vi "getDeviceNameFromDevice.vi"(0 "Controller in":refnum<class "_Controller.lvclass">, 5 "error in (no error)":errorcluster) -> (14 "Controller out":refnum<class "_Controller.lvclass">, 16 "device_name (out)":string, 19 "error out":errorcluster)   [LabVIEW 2020, in "classes.lvlib" / "_Controller.lvclass"]
doc: "Retrieve the Device Name directly from the Controller\n\nProduced By:\n\n<B>Kod Integrations, LLC</B>\n4835 Marianne Drive\nMount Airy, MD 21771\nhttp://www.kodintegrations.com\nemail: info@kodintegrations.com\nphone: (240) 687-1288"
uses:
  _Controller.lvclass
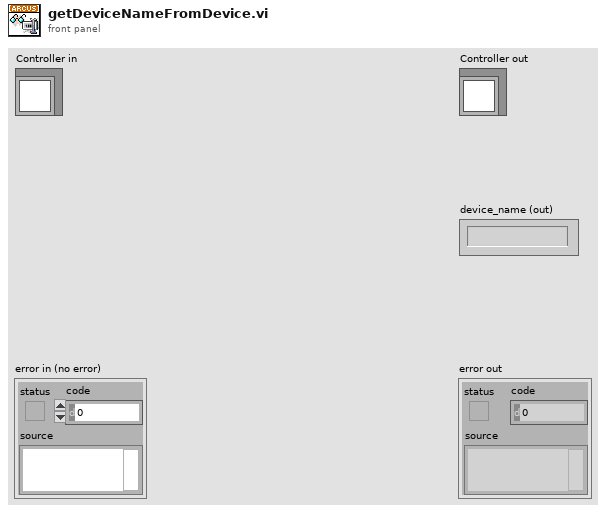
[diagram p1: front panel]
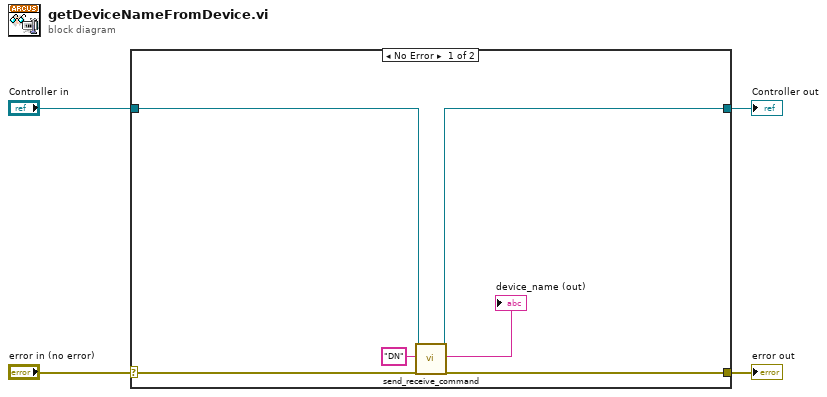
[diagram p0: block diagram]
diagram:
  n1 = case shown="No Error" "error in (no error)" {
    selector: "error in (no error)" -> [w10 w12]
    tunnel: [w9 w12] -> w3
    tunnel: [w6 w11] -> w1
    tunnel: "Controller in" -> [w7 w11]
    frame No Error {
      n2 = call "send_receive_command.vi"("reference (in)"=w7, "ASCII Command (in)"="DN", "error in (no error)"=w10) -> ("reference (out)"=w6:refnum<class "_Controller.lvclass">, "response (out)"=→"device_name (out)":string, "error out"=w9:errorcluster)  [unwired: 12 in, 2 out]
    }
    frame Error {
    }
  }
  "error out" <- w3
  "Controller out" <- w1
